vi "Write Error Cluster Attribute.vi"(9 "JSON value":string, 10 "attribute name":string, 11 "error in":errorcluster) -> (2 "created?":bool, 3 "error out":errorcluster)   [LabVIEW 2020, in "Multi Error Cluster.lvlib"]
doc: "Updates the value of an attribute stored in an error cluster. If the specified attribute name is not found, this VI adds the attribute with the specified value to the error cluster. \n\nFor a single cluster that stores multiple errors, this VI updates only the first error."
uses:
  <vilib>/MultiError/TokenizeJSON/Multi Error Cluster.lvlib
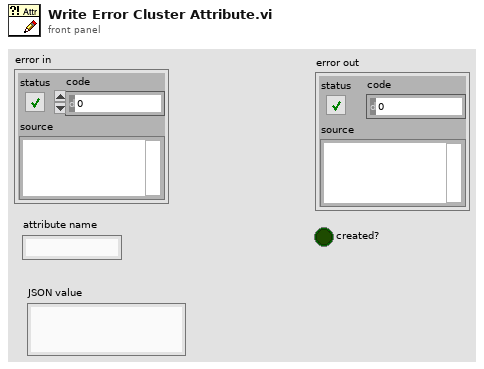
[diagram p1: front panel]
types:
  T1 = typedef "Multi Error Cluster.lvlib/JSON Token Values.ctl" = enum32{"array begin", "array end", "object begin", "object end", "value", "invalid", "name"}
  T2 = typedef "Multi Error Cluster.lvlib/JSON Token Descriptor.ctl" = cluster{"match string":string, "raw token type":T3, "byte offset ":i32}
  T3 = typedef "Multi Error Cluster.lvlib/JSON Raw Token Values.ctl" = enum32{"{", "}", "[", "]", ",", ":", "\"", "number", "string", "true", "false", "null", "invalid"}
  T4 = typedef "Multi Error Cluster.lvlib/JSON Object Descriptor.ctl" = cluster{"begin info":T2, "end info":T2, "begin Index":i32, "end Index":i32}
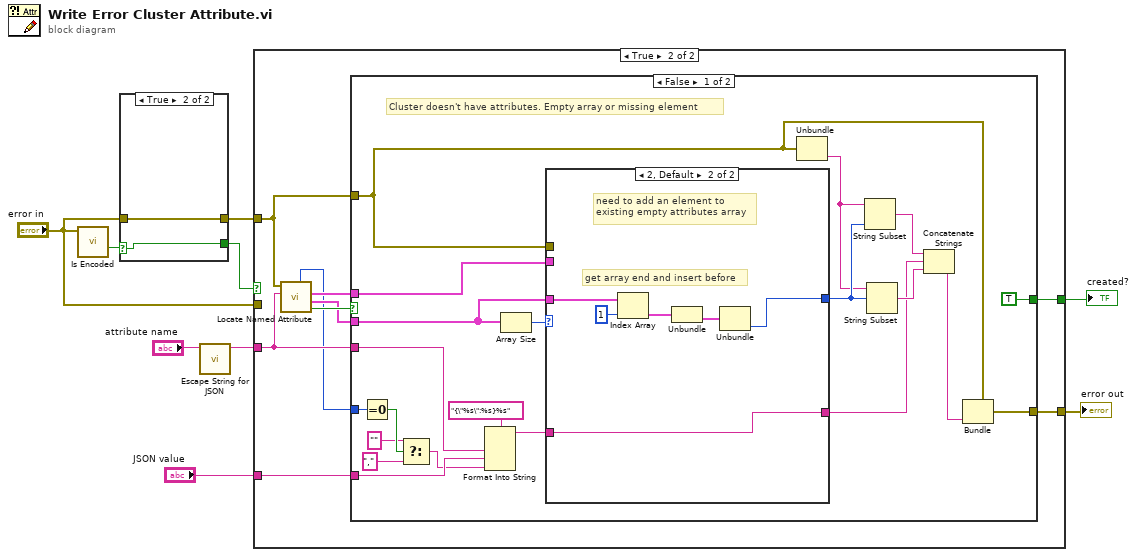
[diagram p0: block diagram]
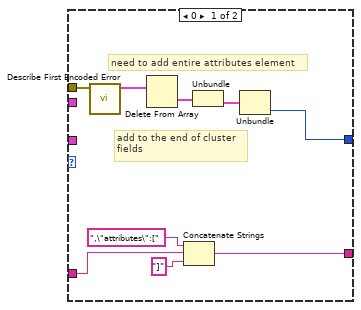
[diagram p3: hidden frame]
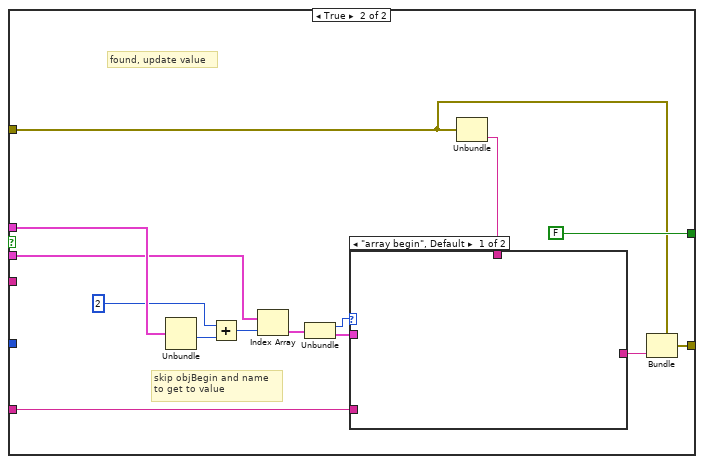
[diagram p4: hidden frame]
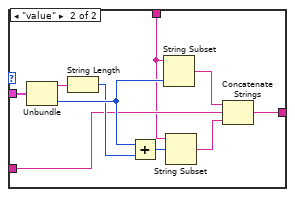
[diagram p5: hidden frame]
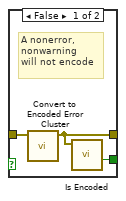
[diagram p6: hidden frame]
diagram:
  n1 = call <vilib>:"Is Encoded.vi"("error in (no error)"="error in") -> ("Is Encoded"=w6:bool)  [unwired: 8 in, 2 out]
  n2 = case shown="True" w6 {
    selector: w6 -> [_ w13]
    tunnel: "error in" -> [w12 w14]
    tunnel: [w11 w14] -> w5
    tunnel: [w10 w13] -> w4
    frame False {
      # "A nonerror,\nnonwarning\nwill not encode"
      n3 = call <vilib>:"Convert to Encoded Error Cluster.vi"("error in"=w12) -> ("error out"=w11:errorcluster)  [unwired: 10 in]
      n4 = call <vilib>:"Is Encoded.vi"("error in (no error)"=w11) -> ("Is Encoded"=w10:bool)  [unwired: 8 in, 2 out]
    }
    frame True {
    }
  }
  n5 = call <vilib>:"Escape String for JSON.vi"("string"="attribute name") -> ("quoted string"=w1:string)  [unwired: 10 in]
  n6 = case shown="True" w4 {
    tunnel: "JSON value" -> [_ w21]
    tunnel: [_ w20] -> w8
    tunnel: [w15 w19] -> w7
    tunnel: w1 -> [_ w18]
    tunnel: w5 -> [_ w17]
    tunnel: "error in" -> [w15 _]
    frame False {
    }
    frame True {
      n7 = call <vilib>:"Locate Named Attribute.vi"("attribute name"=w18, "error"=w17) -> ("found"=w24:bool, "attribute tokens"=w22:cluster{"token type":T1, T2}[], "JSON Object Descriptor"=w23:T4, "attributes"=w16:i32)  [unwired: 5 in, 1 out]
      n8 = case shown="False" w24 {
        tunnel: [TRUE FALSE] -> w20
        tunnel: w17 -> [w26 w63]
        tunnel: w23 -> [w44 w73]
        tunnel: w22 -> [w42 w69]
        tunnel: w21 -> [w35 w65]
        tunnel: [w34 w61] -> w19
        tunnel: w18 -> [w36 _]
        tunnel: w16 -> [w41 _]
        frame False {
          # "Cluster doesn't have attributes. Empty array or missing element"
          n9 = Equal To 0?(x=w41) -> (x = 0?=w39:bool)
          n10 = Select(t="" ("format string"), s=w39, f="," ("format string")) -> (s? t:f=w25:string)
          n11 = Format Into String(format string="{\"%s\":%s}%s", w36, w35, w25) -> (resulting string=w28:string)  [unwired: 2 in, 1 out]
          n12 = Array Size(array=w42) -> (size(s)=w43:i32)
          n13 = case shown="2, Default" w43 {
            tunnel: w44 -> [_ _]
            tunnel: w42 -> [_ w60]
            tunnel: [w46 w57] -> w31
            tunnel: w28 -> [w52 w56]
            tunnel: [w51 w56] -> w27
            tunnel: w26 -> [w50 _]
            frame 0 {
              # "add to the end of cluster\nfields"
              # "need to add entire attributes element"
              n14 = call <vilib>:"Describe First Encoded Error.vi"("error in"=w50) -> ("tokens"=w49:cluster{"token type":T1, T2}[])  [unwired: 9 in, 1 out]
              n15 = Delete From Array(array=w49) -> (deleted portion=w48:cluster{"token type":T1, T2})  [unwired: 2 in, 1 out]
              n16 = Concatenate Strings(",\"attributes\":[" ("format string"), w52, "]" ("format string")) -> (w51:string)
              n17 = Unbundle(w48) -> (w47:T2)  [unwired: 1 out]
              n18 = Unbundle(w47) -> ("byte offset"=w46:i32)  [unwired: 2 out]
            }
            frame 2, Default {
              # "get array end and insert before"
              # "need to add an element to\nexisting empty attributes array"
              n19 = Index Array(array=w60, index=1) -> (element=w59:cluster{"token type":T1, T2})
              n20 = Unbundle(w59) -> (w58:T2)  [unwired: 1 out]
              n21 = Unbundle(w58) -> ("byte offset"=w57:i32)  [unwired: 2 out]
            }
          }
          n22 = Unbundle(w26) -> ("source"=w29:string)  [unwired: 2 out]
          n23 = String Subset(string=w29, length (rest)=w31) -> (substring=w32:string)  [unwired: 1 in]
          n24 = String Subset(string=w29, offset (0)=w31) -> (substring=w33:string)  [unwired: 1 in]
          n25 = Concatenate Strings(w32, w27, w33) -> (w30:string)
          n26 = Bundle(cluster=w26, "source"=w30) -> (w34:errorcluster)  [unwired: 2 in]
        }
        frame True {
          # "skip objBegin and name\nto get to value"
          # "found, update value"
          n27 = Unbundle(w73) -> ("begin Index"=w72:i32)  [unwired: 3 out]
          n28 = Add(x=2, y=w72) -> (x+y=w70:i32)
          n29 = Index Array(array=w69, index=w70) -> (element=w68:cluster{"token type":T1, T2})
          n30 = Unbundle(w68) -> ("token type"=w66:T1, w67:T2)
          n31 = Unbundle(w63) -> ("source"=w64:string)  [unwired: 2 out]
          n32 = case shown="\"array begin\", Default" w66 {
            tunnel: w67 -> [_ w84]
            tunnel: w65 -> [_ w77]
            tunnel: [_ w76] -> w62
            tunnel: w64 -> [_ w75]
            frame "array begin", Default {
            }
            frame "value" {
              n33 = Unbundle(w84) -> ("match string"=w83:string, "byte offset"=w82:i32)  [unwired: 1 out]
              n34 = String Length(string=w83) -> (length=w81:i32)
              n35 = Add(x=w82, y=w81) -> (x+y=w80:i32)
              n36 = String Subset(string=w75, length (rest)=w82) -> (substring=w79:string)  [unwired: 1 in]
              n37 = String Subset(string=w75, offset (0)=w80) -> (substring=w78:string)  [unwired: 1 in]
              n38 = Concatenate Strings(w79, w77, w78) -> (w76:string)
            }
          }
          n39 = Bundle(cluster=w63, "source"=w62) -> (w61:errorcluster)  [unwired: 2 in]
        }
      }
    }
  }
  "error out" <- w7
  "created?" <- w8
